vi "全局变量.vi"() -> ()   [LabVIEW 2011]
panel:
  in  "单选按钮":enum32{"单选选项1", "单选选项2"}(radio)
  in  "报 告 设  置":T1
  in  "采集设置":cluster{"存储路径":path, "Device":u32, "采集间隔时间":u16}={"存储路径"=path "D:/", "Device"=0, "采集间隔时间"=100} {"采集间隔时间" min=200 max=10000 step=100}
  out "提示":string="硬件不存在"
  out "DI":bool[](array[boolean])
  out "DO":bool[](array[boolean])
  in  "卡改变":bool
  in  "选项卡控件":enum32{"采集卡参数", "传感器参数", "任务参数", "报警与控制"}(tab)
  in  "采集卡参数":T2={"量程"="10V", "采集卡类型"="", "端口号"="", "baud rate"=9600, "卡号"="\u0001"}
  in  "传感器参数":string[][](table)=[["通道0", "0", "1", "度"], ["通道1", "0", "1", "度"], ["通道2", "0", "1", "度"], ["通道3", "0", "1", "度"], ["通道4", "0", "1", "度"], ["通道5", "0", "1", "度"], ["通道6", "0", "1", "度"], ["通道7", "0", "1", "度"], ["通道8", "0", "1", "V"], ["通道9", "0", "1", "V"], ["通道10", "0", "1", "V"], ["通道11", "0", "1", "V"], ["通道12", "0", "1", "V"], ["通道13", "0", "1", "V"], ["通道14", "0", "1", "V"], ["通道15", "0", "1", "V"]]
  in  "任务参数":T3={"布尔"=FALSE, "存储路径"=path "D:/", "项目信息"={"项目名称"="", "样品编号"="", "型号规格"="", "检验类型"="", "生产单位"="", "测  试 人"="", "核  对 人"=""}, "时间间隔ms"=0.0, "单帧采样数"=10.0, "自动存储"=FALSE}
  in  "报警与控制参数":T4
  out "频率数据":dbl[](array[numeric])
  out "CNT数据":dbl[](array[numeric])
  in  "量程":string(combo)="10V"
  in  "采集卡类型":string(combo)
  in  "通道数":u8=2 min=2
  in  "精度":dbl
  out "AI数据":dbl[][](array[numeric])
  in  "卡状态":bool
  in  "全体退出":bool
  # "系数设置：例如4-20mA的0-100度温度传感器，则零点设置4，系数设置100/16=6.25。\n重新设置后，右键->数据操作->当前值设置为默认值，即可保存数据，防止下次打开丢失。\n低速记录模式下，采样长度设置低一点，一般设置32；高速采集长度设置高一些。\n历史数据为了防止内存溢出，软件设置最大记录100000组数据。"
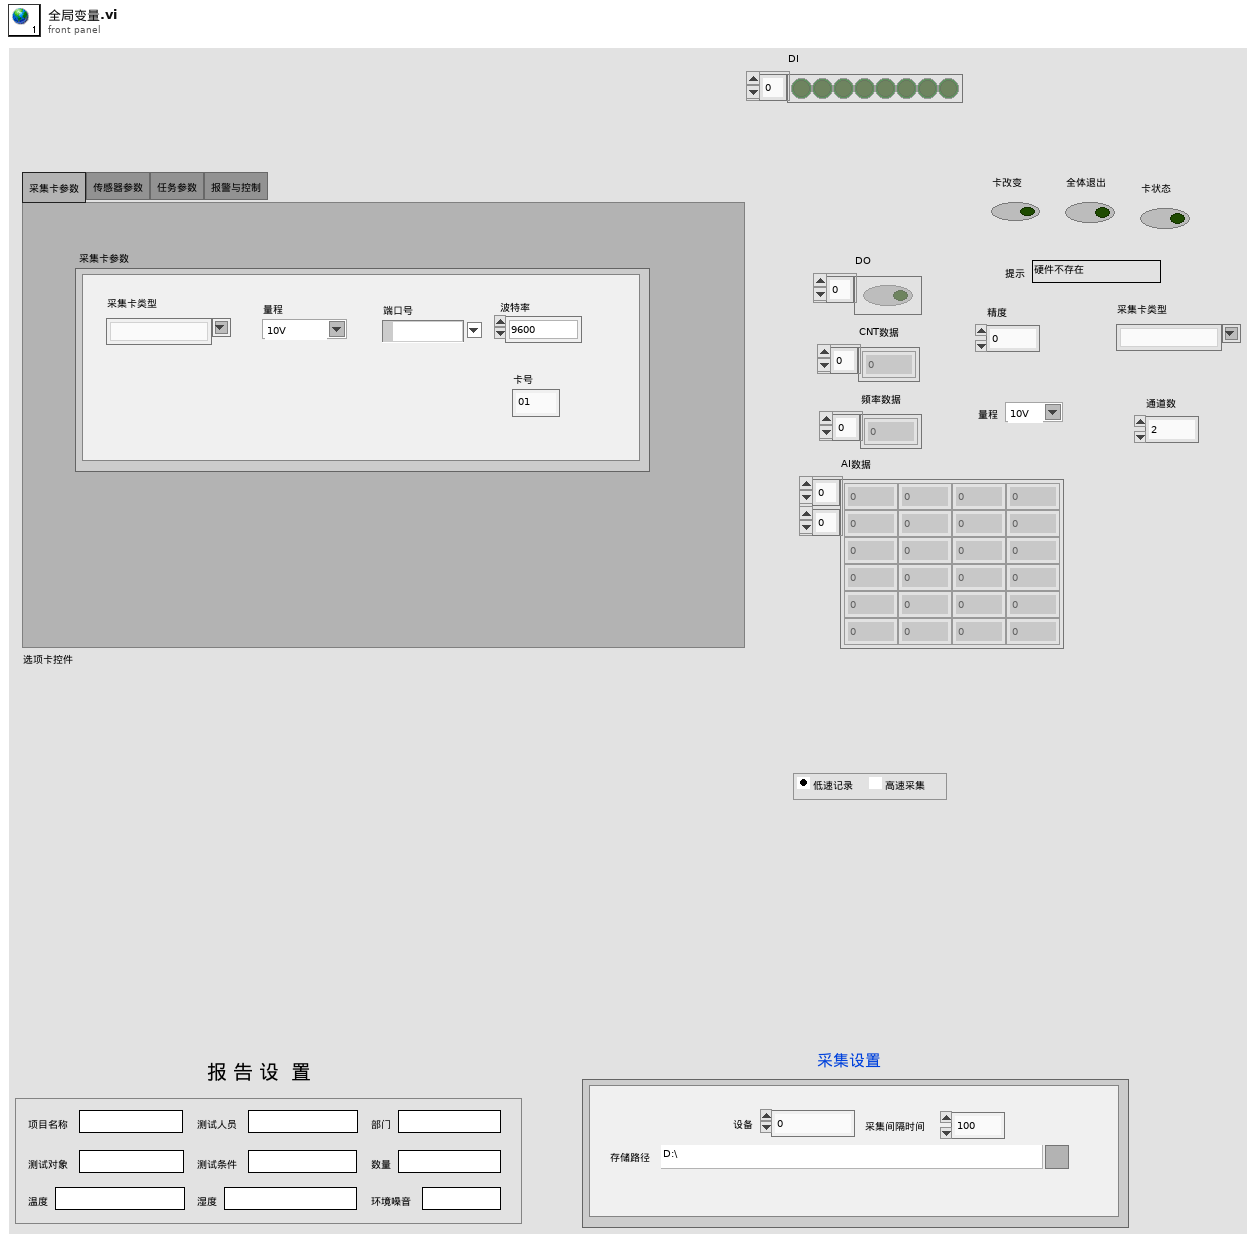
[diagram p1: front panel]
types:
  T1 = cluster{"测试人员":string, "项目名称":string, "部门":string, "测试对象":string, "测试条件":string, "数量":string, "温度":string, "湿度":string, "环境噪音":string}
  T2 = cluster{"量程":string, "采集卡类型":string, "端口号":refnum<visa-resource-name>, "baud rate":u32, "卡号":string}
  T3 = cluster{"布尔":bool, "存储路径":path, "项目信息":cluster{"项目名称":string, "样品编号":string, "型号规格":string, "检验类型":string, "生产单位":string, "测  试 人":string, "核  对 人":string}, "时间间隔ms":dbl, "单帧采样数":dbl, "自动存储":bool}
  T4 = cluster{"事件":string, "类型":string, "通道":string, "服务器IP":string}
diagram:
